vi "cRIO_Host_Cluster_Read_NewMethod_Benchmark.vi"() -> ()   [LabVIEW 2018]
uses:
  TypeDefs/Simple cluster.ctl
  7e8a9f0d-2b7c-4c85-8fb4-747e2fea878c.vi
  7e8a9f0d-2b7c-4c85-8fb4-747e2fea878c.vi/5c86475e-5075-41be-8fd4-ce3a3b6370e5.vi
  FPGA Bitfile Register Operations/Scalar IO Operations/SubVIs/Parse Cluster Configuration.vi
  FPGA Bitfile Register Operations/Scalar IO Operations/Read Methods/Read Data Register/Instances/Read U8 Array.vi
  FPGA Bitfile Register Operations/Scalar IO Operations/SubVIs/Convert Cluster BLOB to Bool Array.vi
  FPGA Bitfile Register Operations/Scalar IO Operations/SubVIs/FXP Raw to DBL.vi
  FPGA Bitfile Register Operations/Scalar IO Operations/FPGA Register IO.lvlib
panel:
  out "error out":errorcluster
  out "Value out":T1
  out "Execution time (s)":dbl
  # "Recorded time"
  # "3.37551E-5"
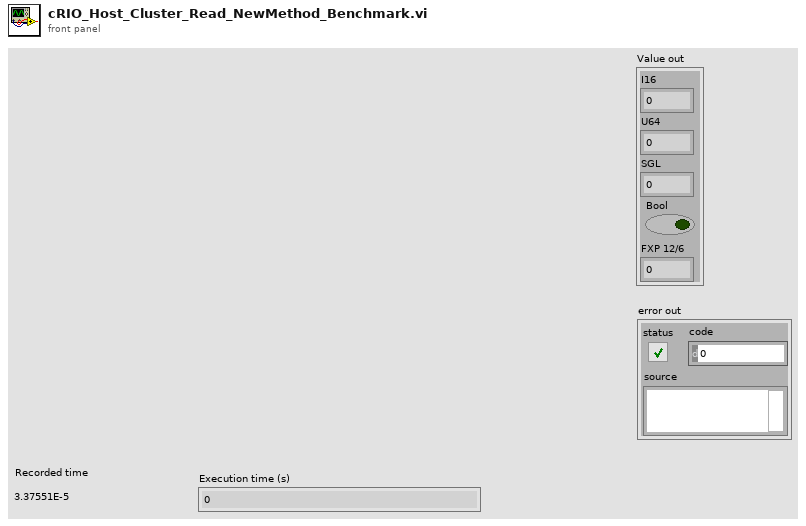
[diagram p1: front panel]
types:
  T1 = typedef "Simple cluster.ctl" = cluster{"I16":i16, "U64":u64, "SGL":sgl, "Bool":bool, "FXP 12/6":fxp<+/-,12,6>}
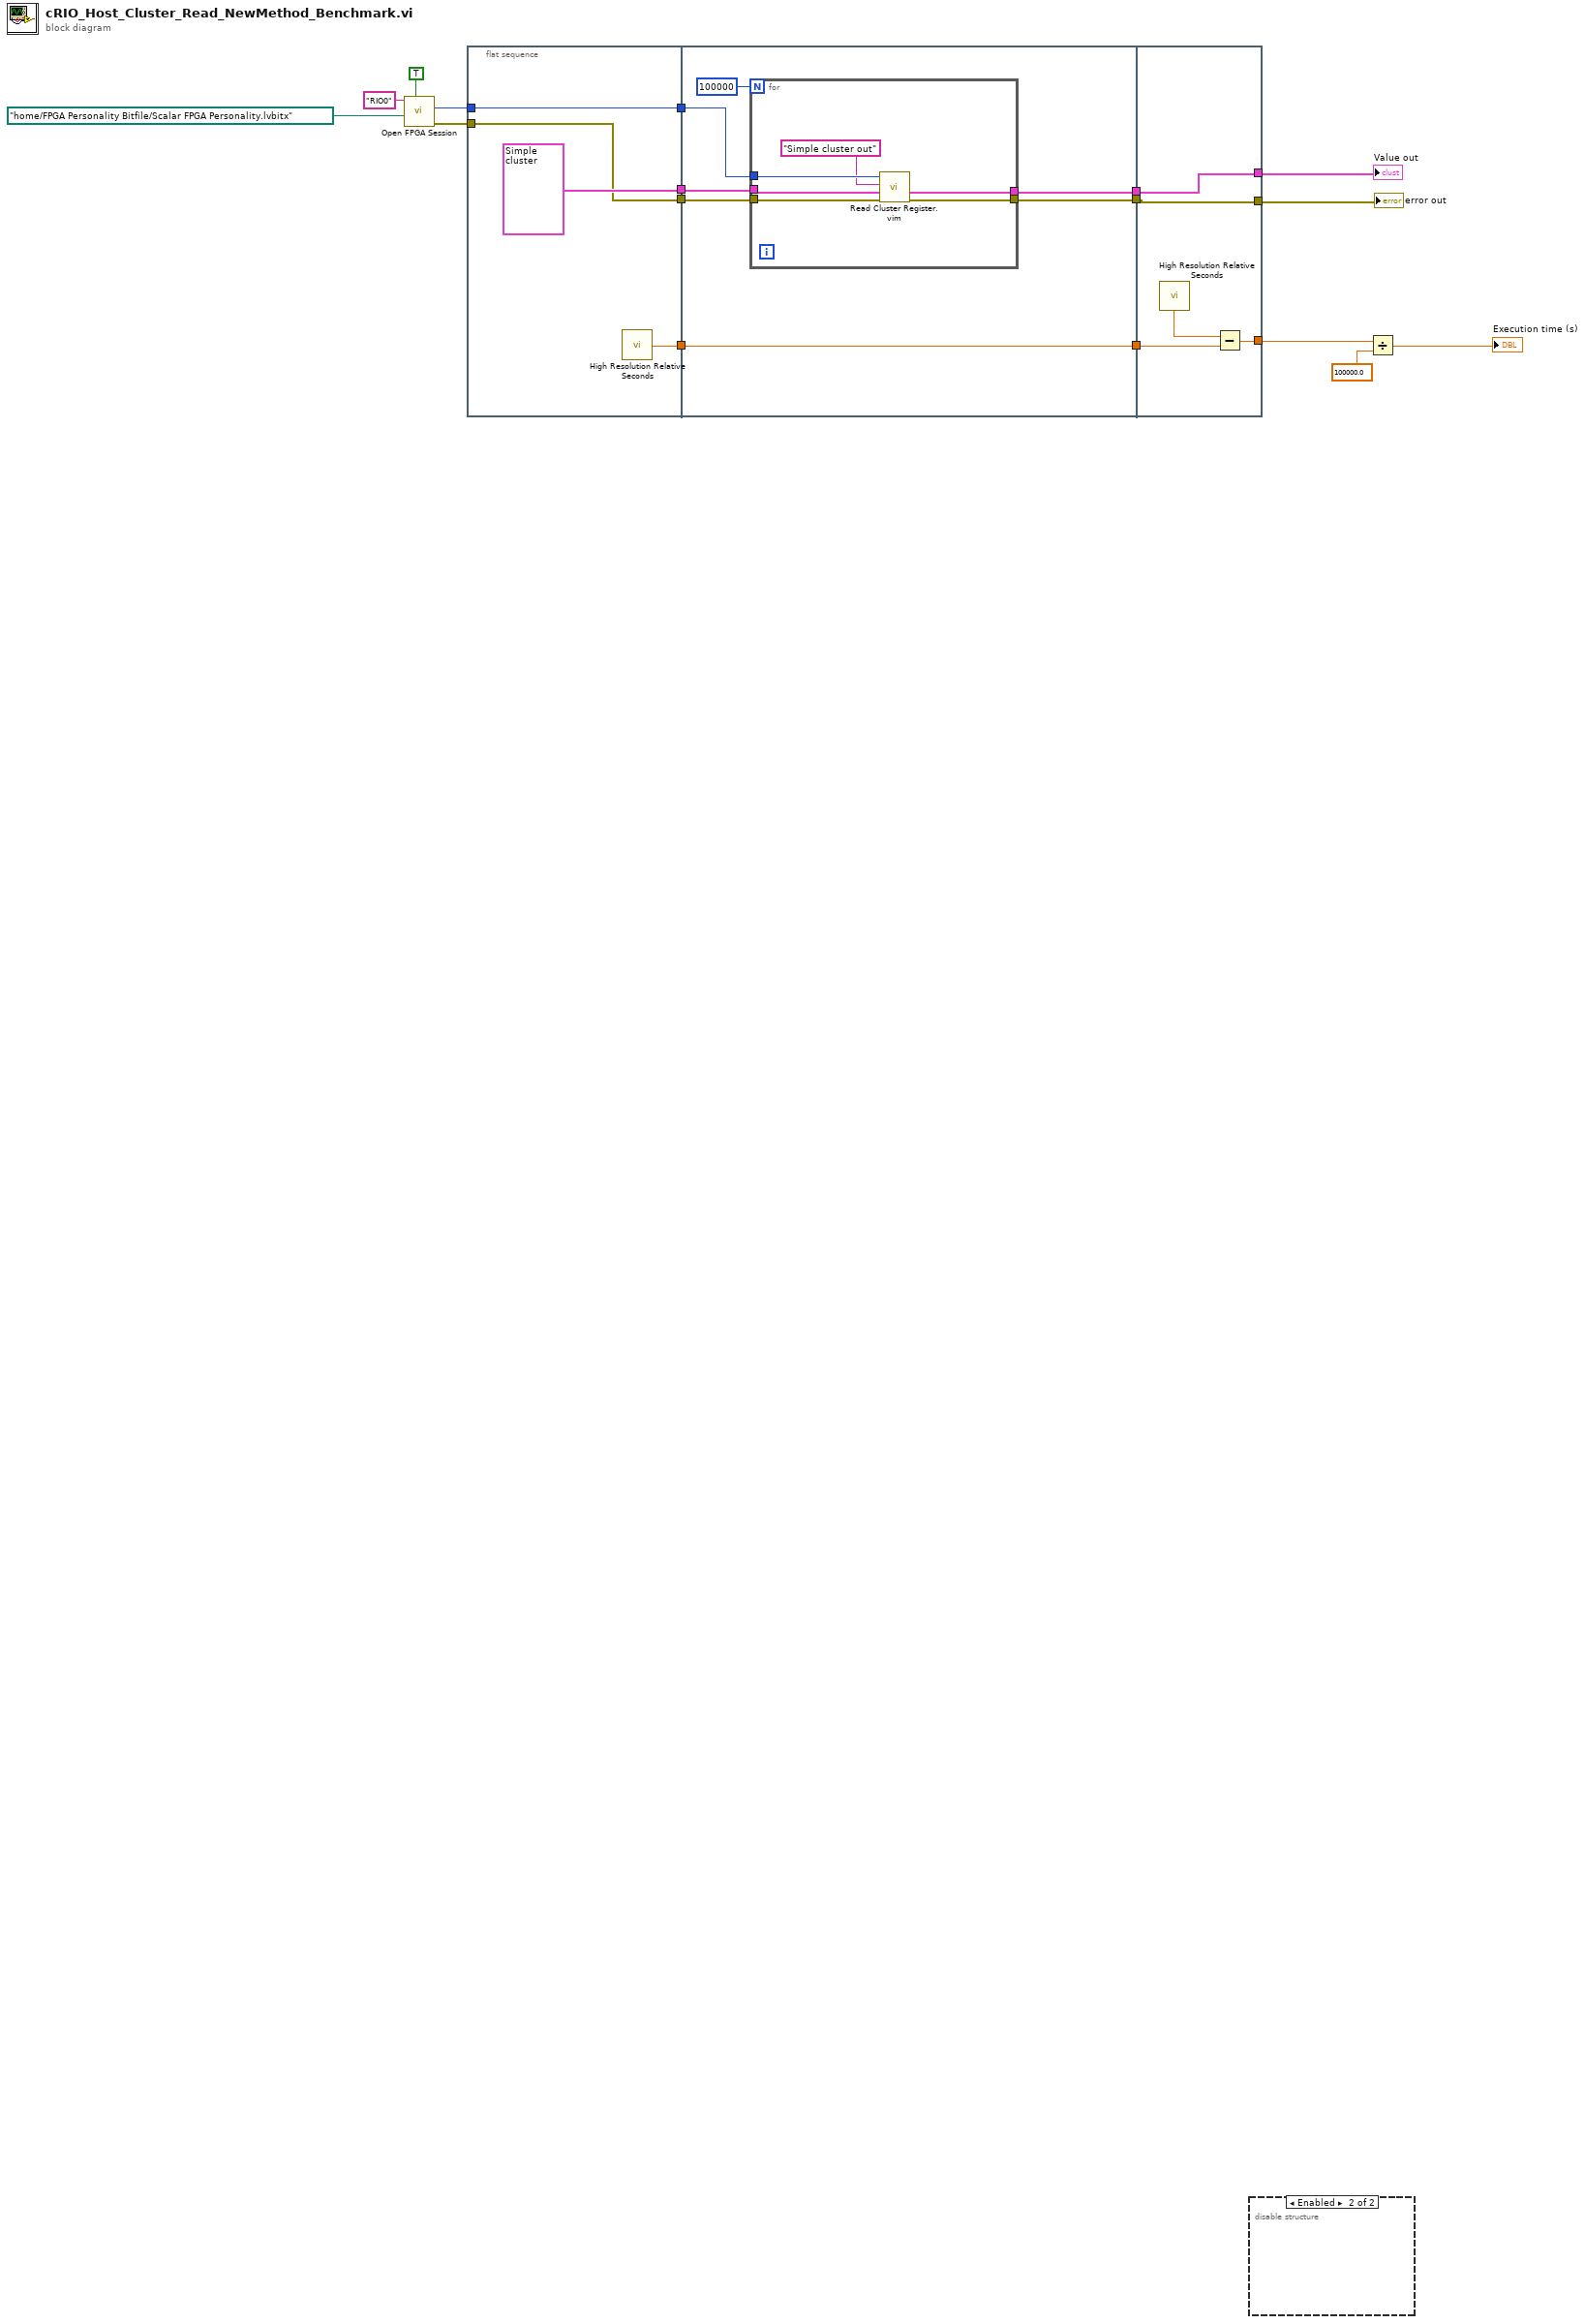
[diagram p0: block diagram]
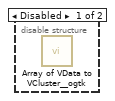
[diagram p2: hidden frame]
diagram:
  n1 = call "Open FPGA Session.vi"("run when loaded (T)"=TRUE, "bitfile path"=path "/home/FPGA Personality Bitfile/Scalar FPGA Personality.lvbitx", "device address"="RIO0") -> ("error out"=w5:errorcluster, "session out"=w10:u32)  [unwired: 6 in, 1 out]
  n2 = flat-sequence {
    tunnel: [T1 {"I16"=1231, "U64"=213123, "SGL"=1.0, "Bool"=TRUE, "FXP 12/6"=31.984375} ("Simple Cluster")] -> w17
    tunnel: [w20] -> w15
    tunnel: w10 -> [w19]
    tunnel: [w19] -> w9
    tunnel: w5 -> [w18]
    tunnel: [w18] -> w4
    tunnel: w17 -> [w27]
    tunnel: [w26] -> w16
    tunnel: w15 -> [w26]
    tunnel: [w25] -> w11
    tunnel: w9 -> [w24]
    tunnel: w4 -> [w23]
    tunnel: [w22] -> w3
    tunnel: w16 -> [w38]
    tunnel: [w37] -> w14
    tunnel: w11 -> [w35]
    tunnel: w3 -> [w36]
    tunnel: [w36] -> w2
    tunnel: [w35] -> w1
    frame #0 {
      n3 = call <vilib>:"High Resolution Relative Seconds.vi"() -> ("relative seconds"=w20:dbl)
    }
    frame #1 {
      n4 = for {
        N: 100000 -> [_]
        tunnel: w27 -> [w32]
        tunnel: [w29] -> w25
        tunnel: w24 -> [w34]
        tunnel: w23 -> [w31]
        tunnel: [w30] -> w22
        n5 = call "Read Cluster Register.vim"("error in (no error)"=w31, "Cluster in (default value)"=w32, "Cluster Name"="Simple cluster out", "session in"=w34) -> ("error out"=w30:errorcluster, "Cluster out"=w29:T1)  [unwired: 5 in, 1 out]
      }
    }
    frame #2 {
      n6 = call <vilib>:"High Resolution Relative Seconds.vi"() -> ("relative seconds"=w39:dbl)
      n7 = Subtract(x=w39, y=w38) -> (x-y=w37:dbl)
    }
  }
  n8 = disable-structure shown="Enabled" {
    frame Disabled {
      n9 = call <userlib>:"Array of VData to VCluster__ogtk.vi"() -> ()  [unwired: 10 in, 2 out]
    }
    frame Enabled {
    }
  }
  n10 = Divide(x=w14, y=100000.0) -> (x/y=→"Execution time (s)":dbl)
  "Value out" <- w1
  "error out" <- w2
